vi "switch_head_tail.vi"(0 "del_in":dbl) -> (1 "del_out":dbl, 2 "rev?":bool)   [LabVIEW 2013]
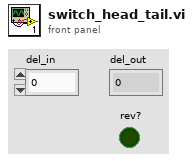
[diagram p1: front panel]
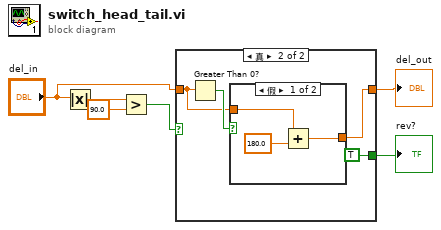
[diagram p0: block diagram]
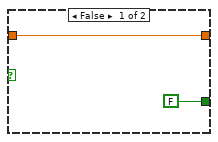
[diagram p2: hidden frame]
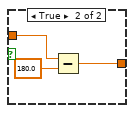
[diagram p3: hidden frame]
diagram:
  n1 = Absolute Value(x="del_in") -> (abs(x)=w4:dbl)
  n2 = Greater?(x=w4, y=90.0) -> (0:w5:bool)
  n3 = case shown="真" w5 {
    tunnel: "del_in" -> [w8 w10]
    tunnel: [w8 w9] -> w3
    tunnel: [FALSE TRUE] -> w2
    frame False {
    }
    frame True {
      n4 = Greater Than 0?(x=w10) -> (x > 0?=w11:bool)
      n5 = case shown="假" w11 {
        tunnel: w10 -> [w15 w17]
        tunnel: [w13 w16] -> w9
        frame False {
          n6 = Add(x=w15, y=180.0) -> (x+y=w13:dbl)
        }
        frame True {
          n7 = Subtract(x=w17, y=180.0) -> (x-y=w16:dbl)
        }
      }
    }
  }
  "del_out" <- w3
  "rev?" <- w2
